vi "Do_channel_maths.vi"(4 "Output Index":i32, 5 "Channel Values In":string[][](array[string]), 6 "Channel Names":string[](array[string]), 7 "Maths Equation":string) -> (0 "Error String":string, 1 "Channel Values Out":string[][](array[string]), 3 "Results":dbl[](array[numeric]) format="%0.2f")   [LabVIEW 2021]
uses:
  Data_plotting_vis/Results_plotter_Global.vi
  <vilib>/gmath/NI_Gmath.lvlib
panel:
  out "Numeric":i32
  out "AuditTrail":string[](array[string])
  out "Generic Equation":string
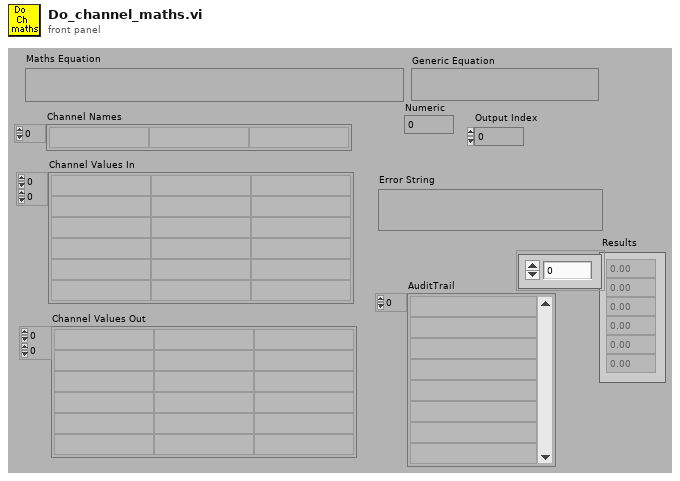
[diagram p1: front panel]
types:
  T1 = cluster{"Tables":i32[][], "Y Values":dbl[], "Variables input decode":i32[], i32[]}[]
  T2 = cluster{"Y Values":dbl[][], "Tables":i32[][][], "Variables input decode":i32[], "Variables output decode":i32[]}
  T3 = cluster{"Tables":i32[][], "Y Values":dbl[], "Variables input decode":i32[], i32[]}
  T4 = typedef "LVDateTimeRec.ctl" = cluster{"fractional second":dbl, "second":i32, "minute":i32, "hour":i32, "day of month":i32, "month":i32, "year":i32, "day of week":i32, "day of year":i32, "DST":i32}
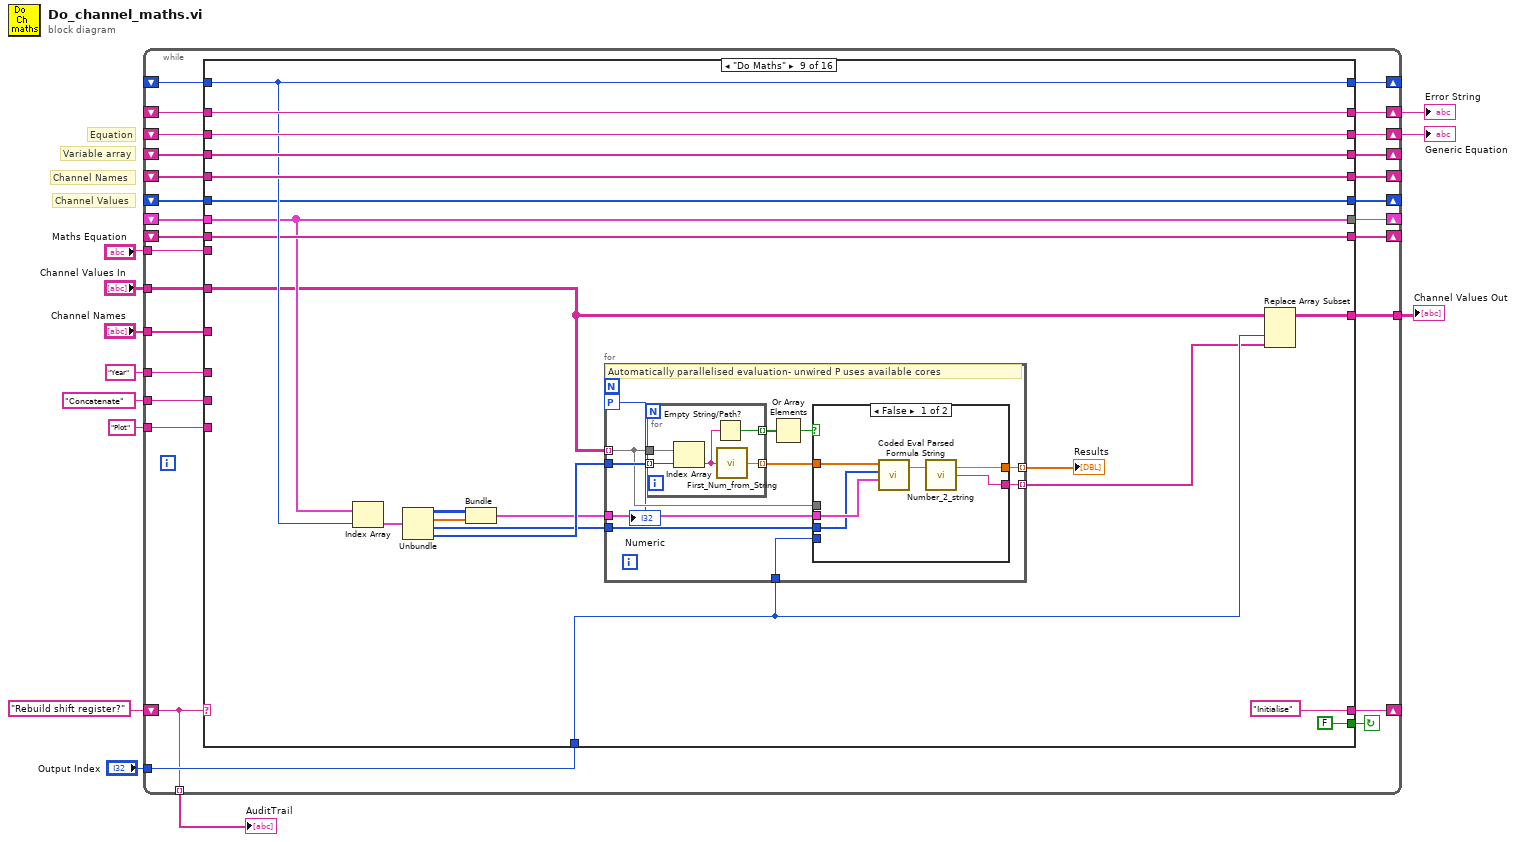
[diagram p0: block diagram]
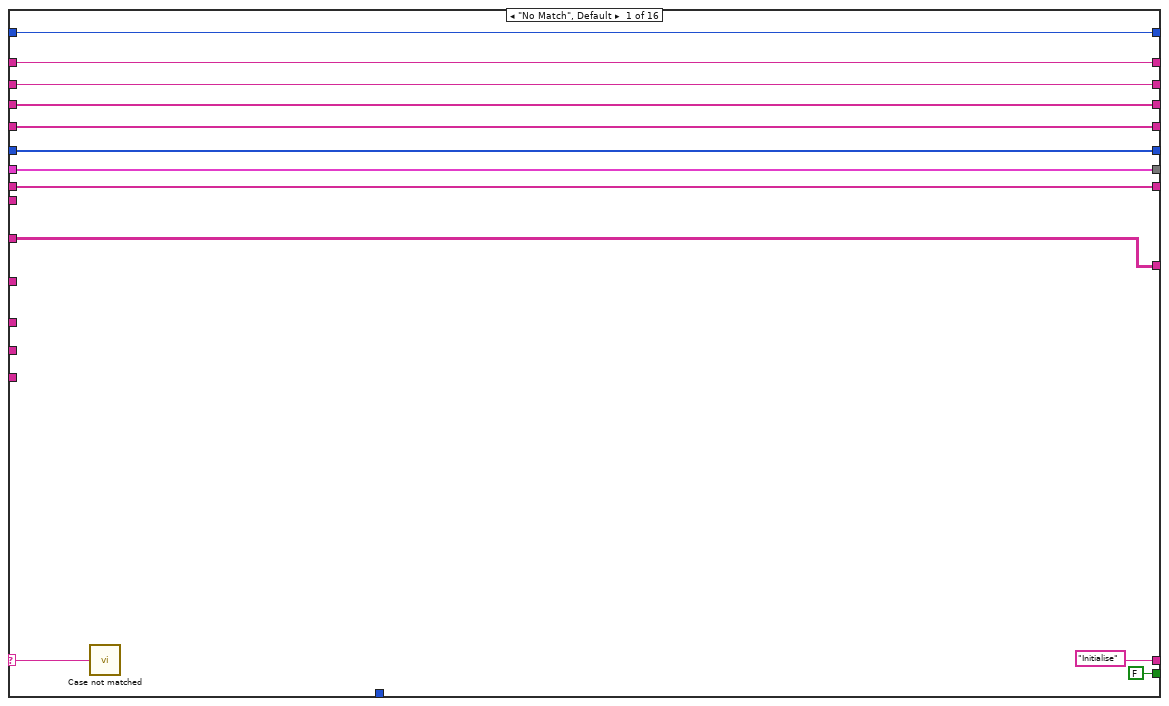
[diagram p2: hidden frame]
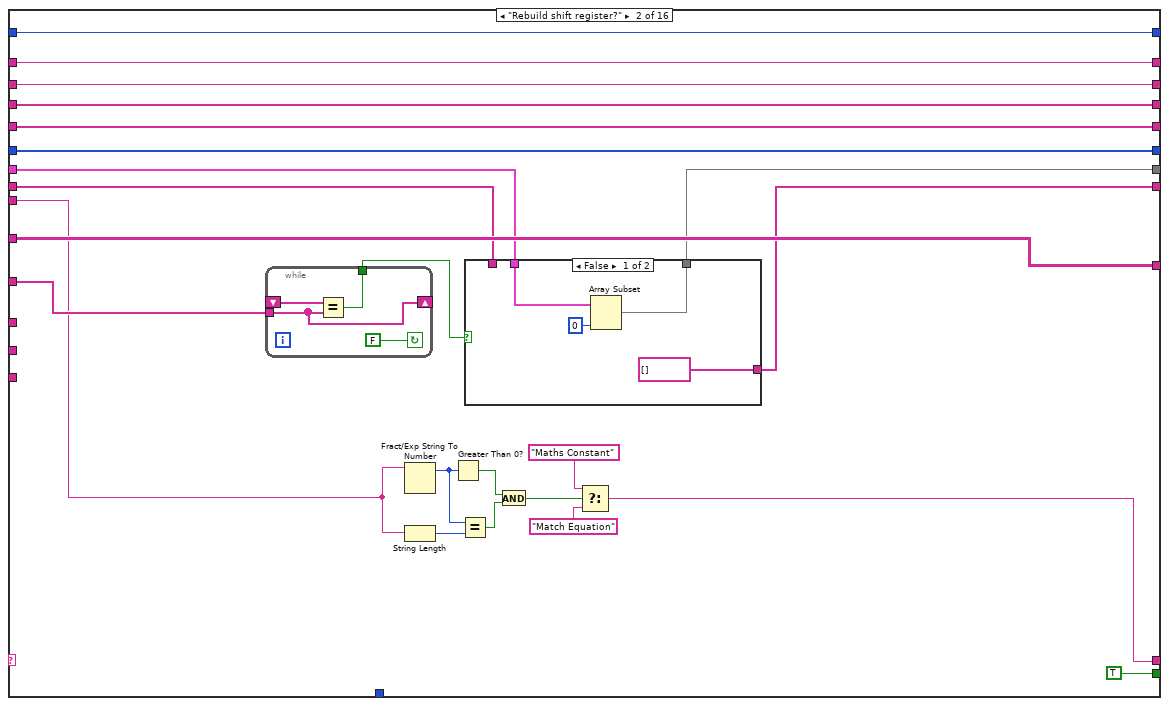
[diagram p3: hidden frame]
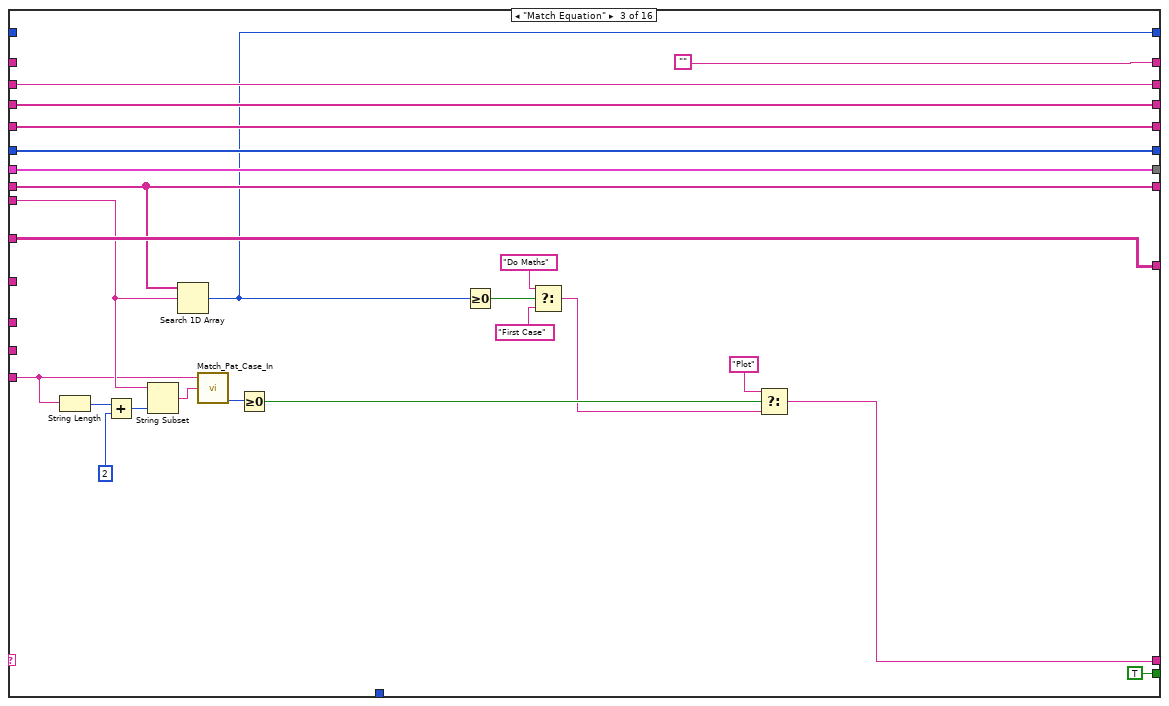
[diagram p5: hidden frame]
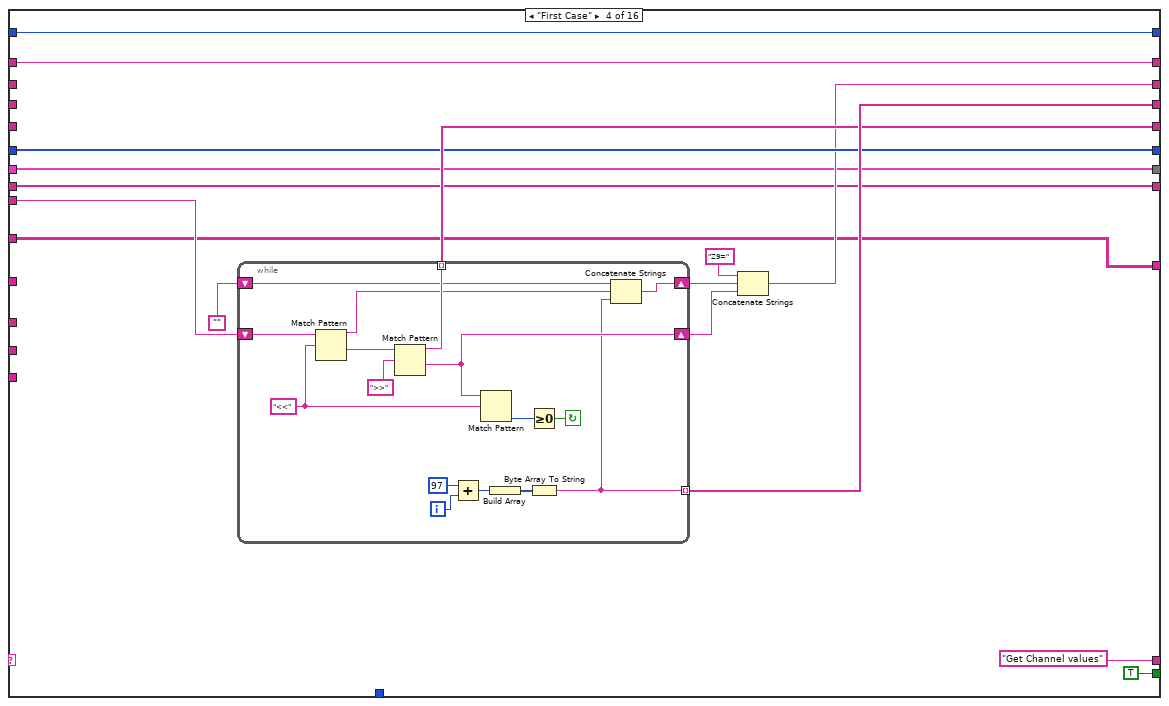
[diagram p6: hidden frame]
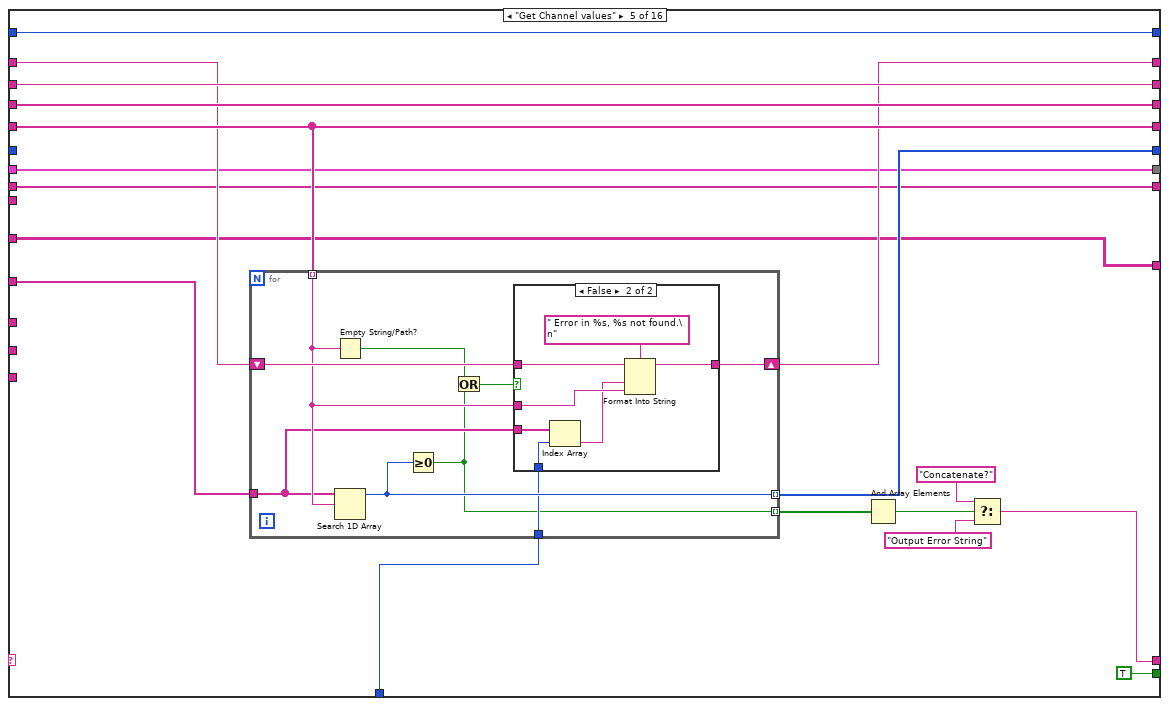
[diagram p7: hidden frame]
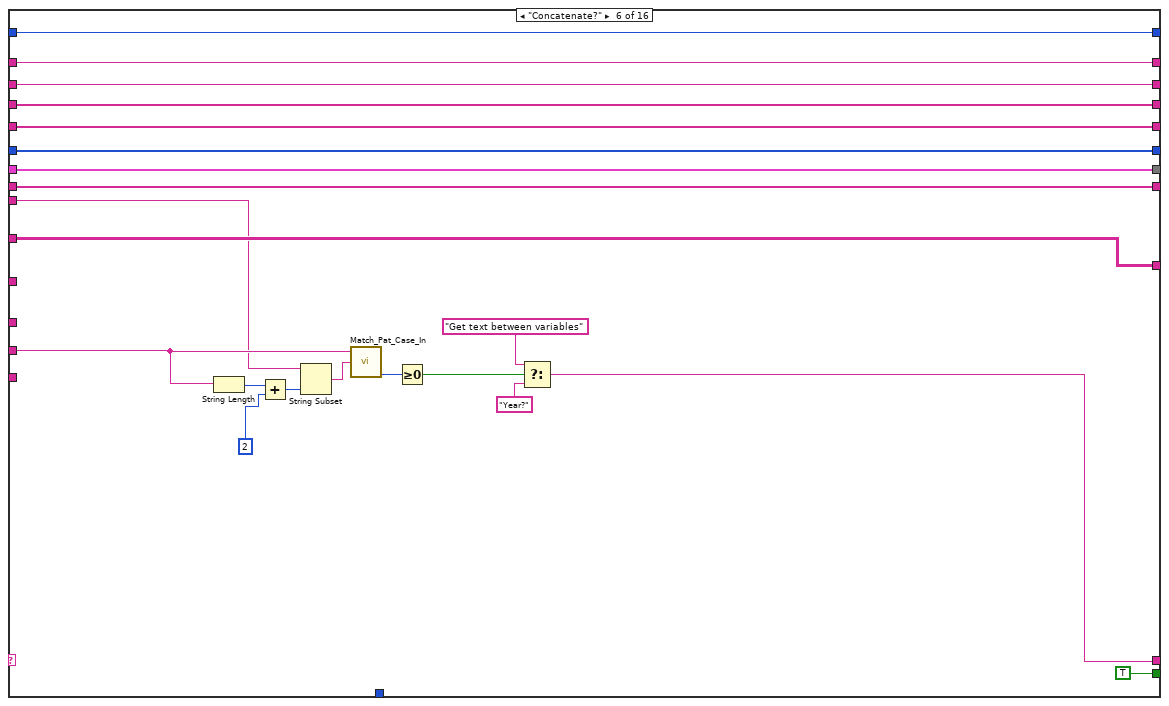
[diagram p9: hidden frame]
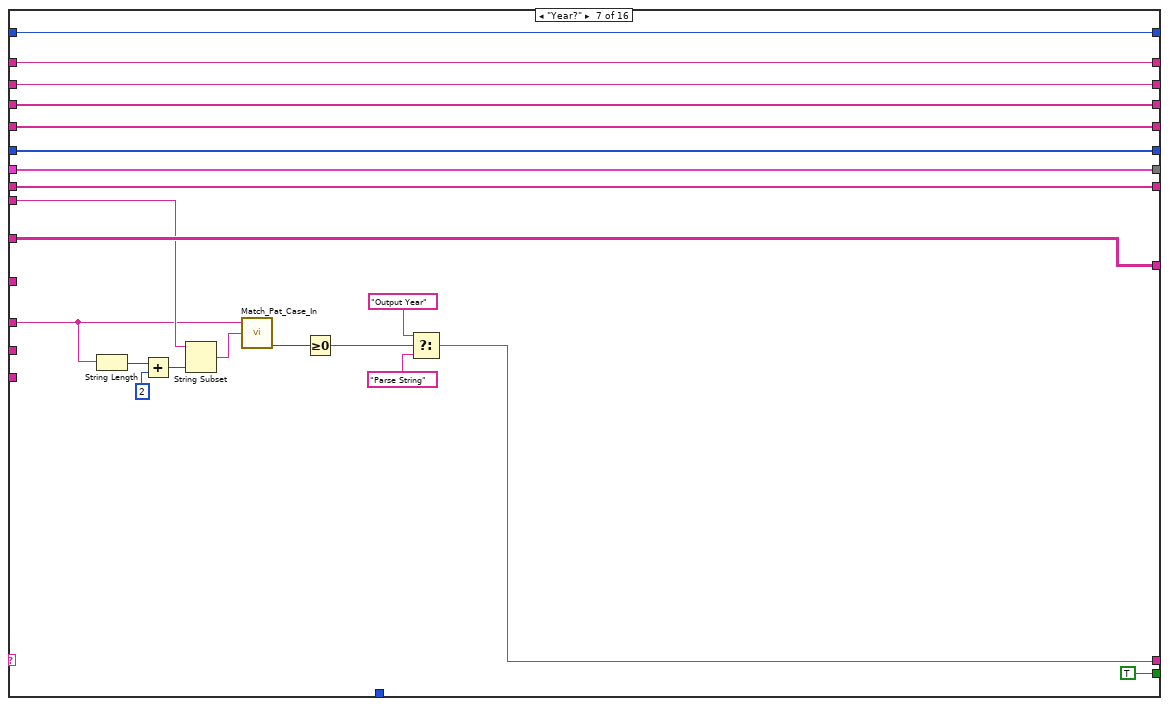
[diagram p10: hidden frame]
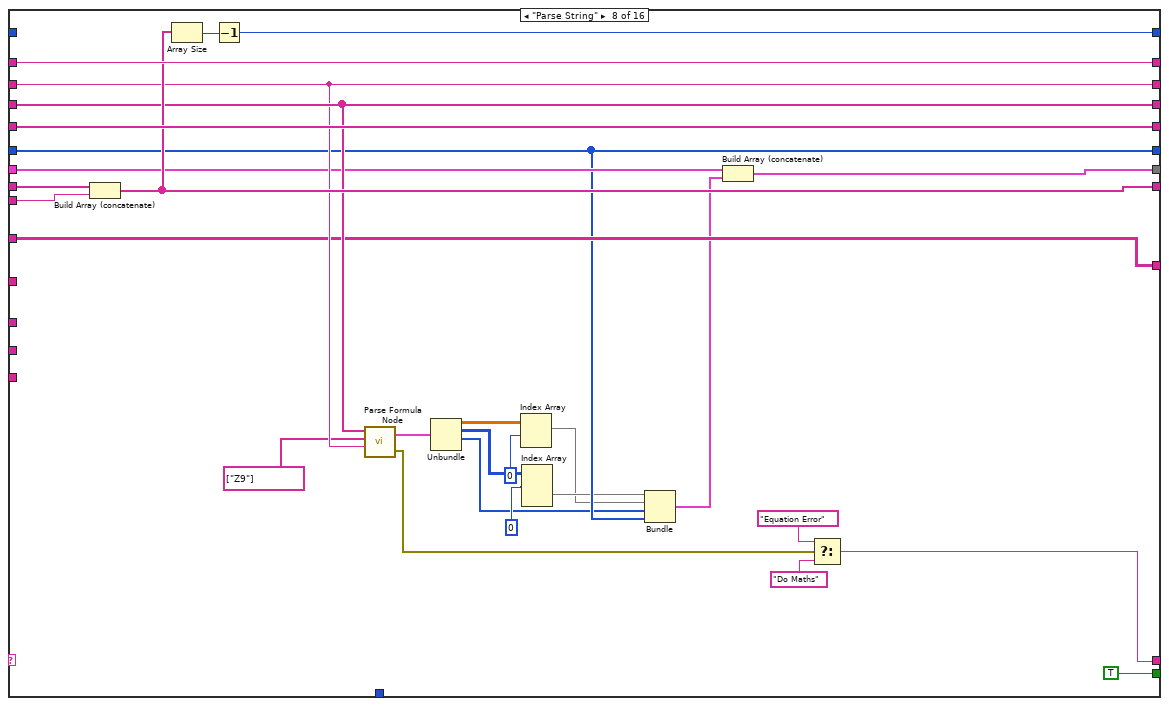
[diagram p11: hidden frame]
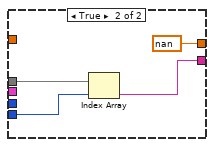
[diagram p12: hidden frame]
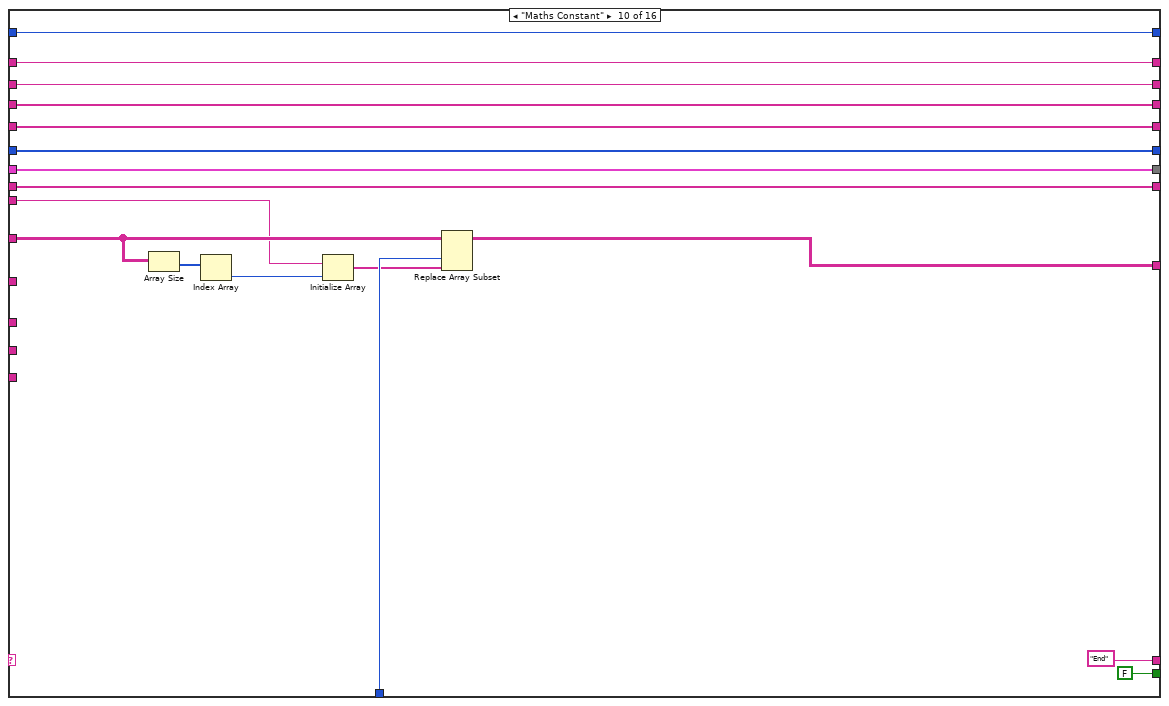
[diagram p13: hidden frame]
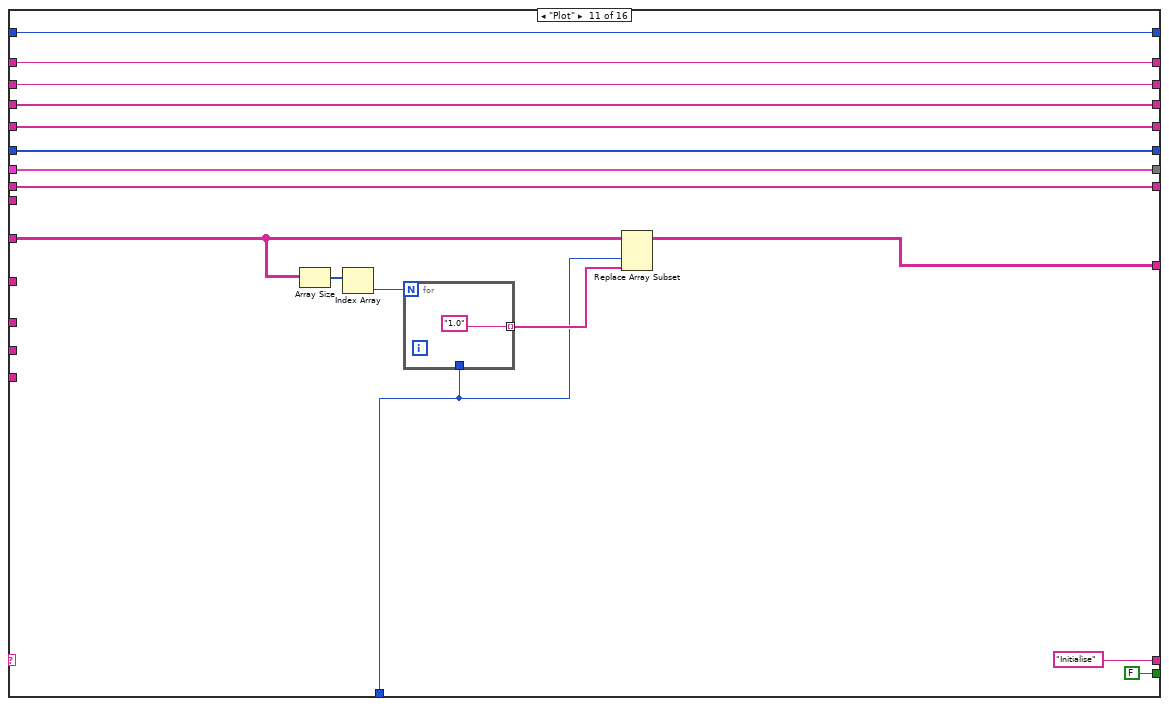
[diagram p14: hidden frame]
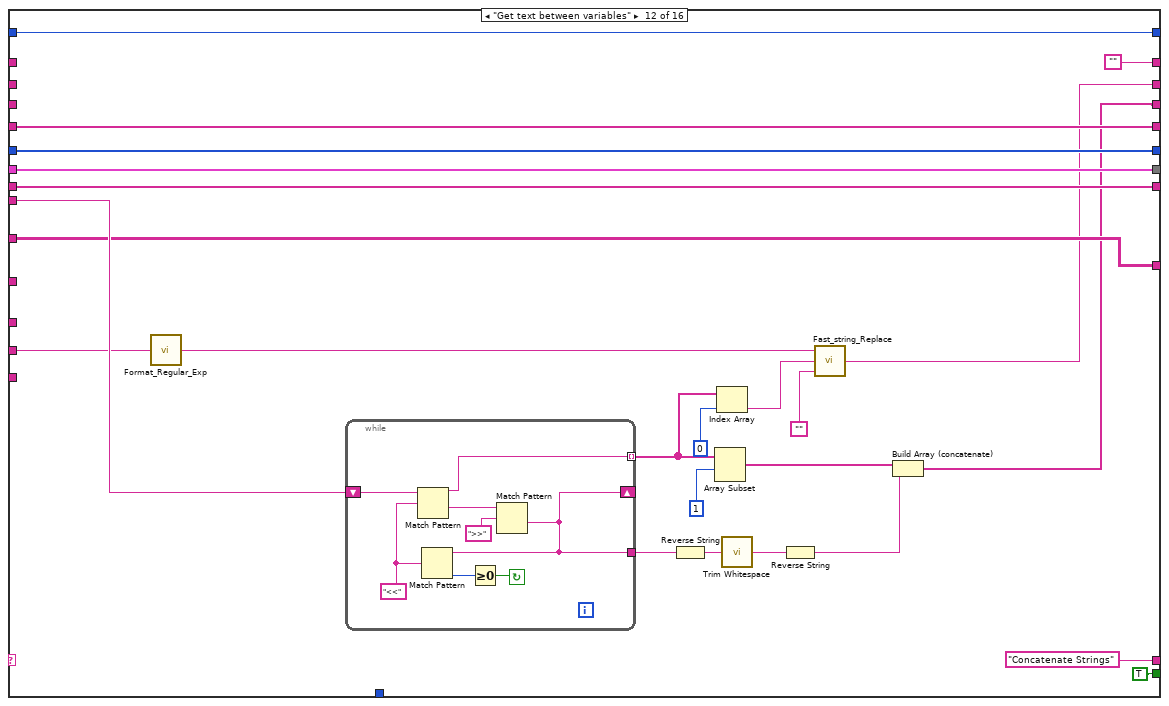
[diagram p15: hidden frame]
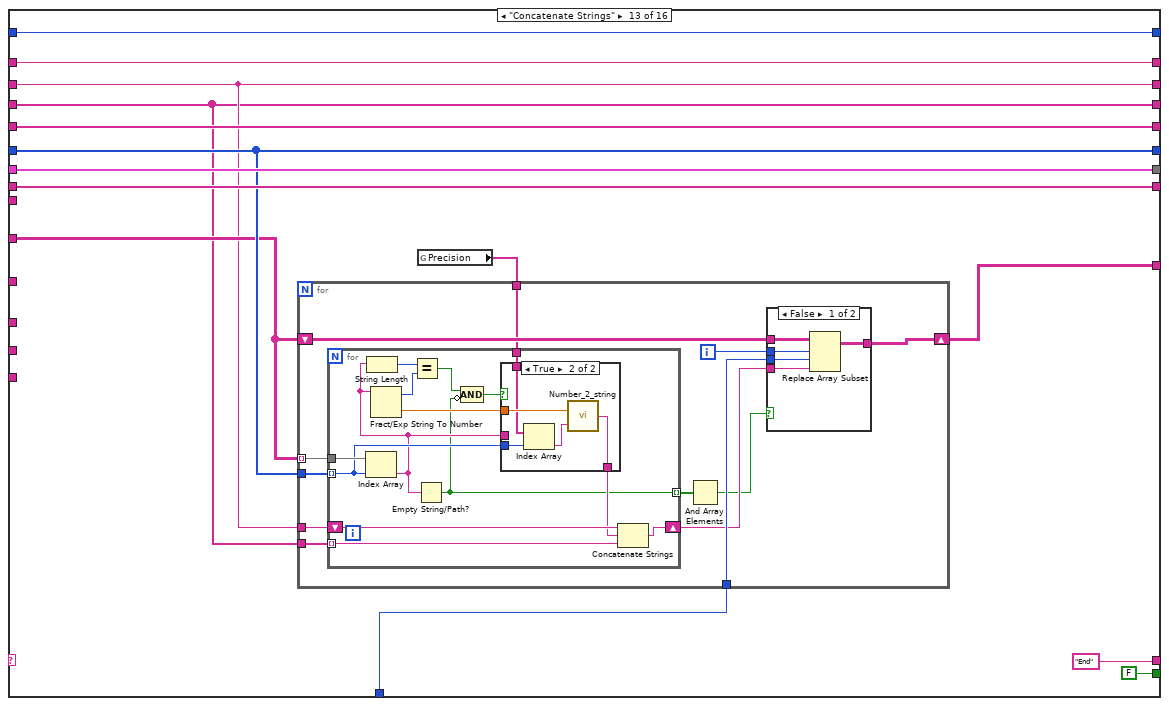
[diagram p16: hidden frame]
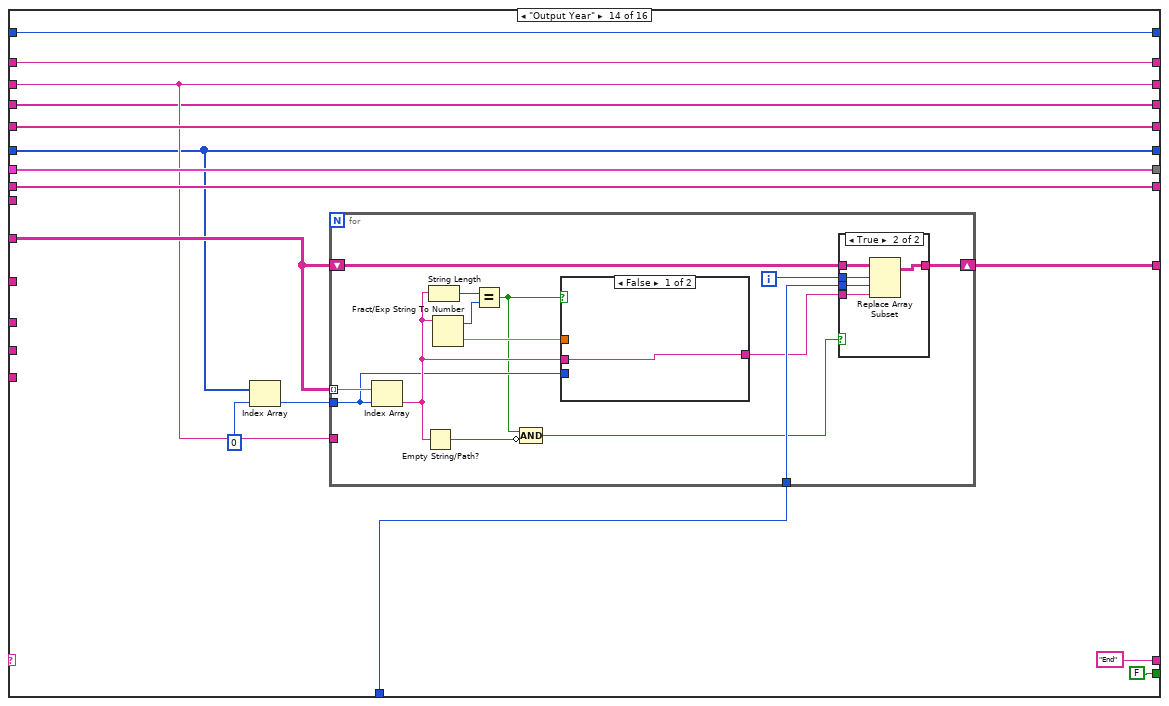
[diagram p19: hidden frame]
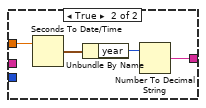
[diagram p20: hidden frame]
diagram:
  # "Channel Names"
  # "Variable array"
  # "Channel Values"
  # "Equation"
  n1 = while {
    tunnel: [w17] -> w6
    tunnel: "Output Index" -> [w18]
    shift-left: _ -> [w19]
    shift-right: [w20] -> _
    shift-left: _ -> [w23]
    shift-right: [w22] -> _
    shift-left: _ -> [w21]
    shift-right: [w24] -> _
    tunnel: "Channel Values In" -> [w25]
    tunnel: "Channel Names" -> [w26]
    tunnel: "Maths Equation" -> [w27]
    shift-left: _ -> [w29]
    shift-right: [w28] -> _
    shift-left: _ -> [w31]
    shift-right: [w30] -> _
    shift-left: _ -> [w33]
    shift-right: [w32] -> _
    shift-left: _ -> [w35]
    shift-right: [w34] -> w8
    shift-left: _ -> [w37]
    shift-right: [w36] -> w9
    shift-left: "Rebuild shift register?" -> [w13]
    shift-right: [w38] -> _
    tunnel: "Concatenate" ("regular expression") -> [w16]
    tunnel: "Plot" ("regular expression") -> [w15]
    tunnel: "Year" ("regular expression") -> [w14]
    tunnel: [w13] -> w1 mode=indexing
    stop <- w39 continue-if-true
    n2 = case shown="\"Do Maths\"" w13 {
      selector: w13 -> [w40 _ _ _ _ _ _ _ _ _ _ _ _ _ _ _]
      tunnel: [FALSE TRUE TRUE TRUE TRUE TRUE TRUE TRUE FALSE FALSE FALSE TRUE FALSE FALSE TRUE FALSE] -> w39
      tunnel: ["Initialise" w53 w86 "Get Channel values" w143 w176 w206 w232 "Initialise" "End" "Initialise" "Concatenate Strings" "End" "End" "Output Error String" "Initialise"] -> w38
      tunnel: w37 -> [w49 w73 _ w109 w151 w196 w217 w243 w263 w305 w321 _ w368 w421 w451 w464]
      tunnel: [w49 w73 "" w109 w152 w196 w217 w243 w263 w305 w321 "" w368 w421 w450 w464] -> w36
      tunnel: w35 -> [w48 w72 w108 _ w157 w195 w216 w239 w261 w303 w319 _ w360 w414 w453 w474]
      tunnel: [w48 w72 w108 w114 w157 w195 w216 w239 w261 w303 w319 w335 w360 w414 w453 w474] -> w34
      tunnel: w33 -> [w47 w71 w107 _ w156 w194 w215 w240 w262 w304 w320 _ w359 w413 w460 w475]
      tunnel: [w47 w71 w107 w121 w156 w194 w215 w240 w262 w304 w320 w330 w359 w413 w460 w475] -> w32
      tunnel: w31 -> [w46 w70 w106 _ w154 w193 w214 w244 w264 w306 w322 w340 w369 w422 w461 w476]
      tunnel: [w46 w70 w106 w117 w154 w193 w214 w244 w264 w306 w322 w340 w369 w422 w461 w476] -> w30
      tunnel: w29 -> [w45 w69 w105 w116 _ w192 w213 w231 w254 w299 w315 w345 w364 w412 w456 w468]
      tunnel: [w45 w69 w105 w116 w153 w192 w213 w231 w254 w299 w315 w345 w364 w412 w456 w468] -> w28
      tunnel: w27 -> [_ w52 w92 w122 _ w180 w200 w218 _ w293 _ w347 _ _ w452 _]
      tunnel: w26 -> [_ w66 _ _ w155 _ _ _ _ _ _ _ _ _ _ w466]
      tunnel: w25 -> [w41 w67 w103 w110 w147 w187 w205 w235 w252 w296 w311 w341 w363 w417 w455 w467]
      tunnel: [w44 w64 w104 w113 w150 w191 w212 w236 w258 w300 w316 w344 w365 w418 w457 w471] -> w24
      tunnel: w23 -> [w43 w62 w102 w112 w149 w190 w211 w242 w259 w301 w317 w343 w366 w419 w458 w472]
      tunnel: [w43 w61 w102 w112 w149 w190 w211 w241 w259 w301 w317 w343 w366 w419 w458 w472] -> w22
      tunnel: w21 -> [w44 w63 w104 w113 w150 w191 w212 w238 w258 w300 w316 w344 w365 w418 w457 w471]
      tunnel: [w42 w68 w101 w111 w148 w189 w210 w237 w260 w302 w318 w342 w367 w420 w459 w473] -> w20
      tunnel: w19 -> [w42 w68 _ w111 w148 w189 w210 _ w260 w302 w318 w342 w367 w420 w459 w473]
      tunnel: w18 -> [_ _ _ _ w141 _ _ _ w251 w297 w312 _ w362 w416 _ w470]
      tunnel: [w41 w67 w103 w110 w147 w187 w205 w235 w253 w298 w314 w341 w361 w415 w455 w469] -> w17
      tunnel: w16 -> [_ _ _ _ _ w186 _ _ _ _ _ w337 _ _ _ _]
      tunnel: w15 -> [_ _ w91 _ _ _ _ _ _ _ _ _ _ _ _ _]
      tunnel: w14 -> [_ _ _ _ _ _ w197 _ _ _ _ _ _ _ _ _]
      frame "No Match", Default {
        n3 = call "Case not matched.vi"("Case Name not Matched"=w40) -> ()
      }
      frame "Rebuild shift register?" {
        n4 = while {
          shift-right: [w83] -> _
          shift-left: _ -> [w84]
          tunnel: w66 -> [w83]
          tunnel: [w82] -> w65
          stop <- FALSE continue-if-true
          n5 = Equal?(x=w84, y=w83) -> (x = y?=w82:bool)
        }
        n6 = Fract/Exp String To Number(string=w52) -> (offset past number=w60:i32)  [unwired: 3 in, 1 out]
        n7 = String Length(string=w52) -> (length=w59:i32)
        n8 = Greater Than 0?(x=w60) -> (x > 0?=w57:bool)
        n9 = Equal?(x=w60, y=w59) -> (x = y?=w58:bool)
        n10 = case shown="False" w65 {
          tunnel: [w76 w80] -> w64
          tunnel: w63 -> [w78 w80]
          tunnel: w62 -> [_ w79]
          tunnel: [string[] [] w79] -> w61
          frame False {
            n11 = Array Subset(array=w78, length=0) -> (w76:T1)  [unwired: 1 in]
          }
          frame True {
          }
        }
        n12 = And(x=w57, y=w58) -> (x .and. y?=w56:bool)
        n13 = Select(t="Maths Constant", s=w56, f="Match Equation") -> (s? t:f=w53:string)
      }
      frame "Match Equation" {
        n14 = String Length(string=w91) -> (length=w93:i32)
        n15 = Add(x=w93, y=2) -> (x+y=w95:i32)
        n16 = String Subset(string=w92, length (rest)=w95) -> (substring=w96:string)  [unwired: 1 in]
        n17 = Search 1D Array(1D array=w102, element=w92) -> (index of element=w101:i32)  [unwired: 1 out]
        n18 = call "Match_Pat_Case_In.vi"("String to match"=w91, "String"=w96) -> ("offset past match"=w89:i32)  [unwired: 1 in, 3 out]
        n19 = Greater Or Equal To 0?(x=w89) -> (x >= 0?=w88:bool)
        n20 = Greater Or Equal To 0?(x=w101) -> (x >= 0?=w100:bool)
        n21 = Select(t="Do Maths", s=w100, f="First Case") -> (s? t:f=w87:string)
        n22 = Select(t="Plot", s=w88, f=w87) -> (s? t:f=w86:string)
      }
      frame "First Case" {
        n23 = while {
          shift-left: "" -> [w127]
          shift-right: [w128] -> w119
          tunnel: [w129] -> w121 mode=indexing
          tunnel: [w135] -> w117 mode=indexing
          shift-left: w122 -> [w140]
          shift-right: [w138] -> w118
          i -> [w131]
          stop <- w136 continue-if-true
          w126 = "<<" ("regular expression")
          n24 = Match Pattern(string=w140, regular expression=w126) -> (before substring=w130:string, after substring=w139:string)  [unwired: 3 out]
          n25 = Match Pattern(string=w139, regular expression=">>") -> (before substring=w135:string, after substring=w138:string)  [unwired: 3 out]
          n26 = Add(x=97, y=w131) -> (x+y=w133:i32)
          n27 = Match Pattern(string=w138, regular expression=w126) -> (offset past match=w137:i32)  [unwired: 4 out]
          n28 = Build Array(w133) -> (w134:i32[])
          n29 = Greater Or Equal To 0?(x=w137) -> (x >= 0?=w136:bool)
          n30 = Byte Array To String(unsigned byte array=w134) -> (string=w129:string)
          n31 = Concatenate Strings(w127, w130, w129) -> (w128:string)
        }
        n32 = Concatenate Strings("Z9=" ("Substring"), w119, w118) -> (w114:string)
      }
      frame "Get Channel values" {
        n33 = for {
          tunnel: w155 -> [w162]
          tunnel: w154 -> [w164] mode=indexing
          tunnel: [w165] -> w153 mode=indexing
          shift-right: [w166] -> w152
          shift-left: w151 -> [w167]
          tunnel: [w159] -> w146 mode=indexing
          tunnel: w141 -> [w161]
          n34 = Empty String/Path?(string/path=w164) -> (empty?=w160:bool)
          n35 = Search 1D Array(1D array=w162, element=w164) -> (index of element=w165:i32)  [unwired: 1 out]
          n36 = Greater Or Equal To 0?(x=w165) -> (x >= 0?=w159:bool)
          n37 = Or(x=w160, y=w159) -> (x .or. y?=w163:bool)
          n38 = case shown="False" w163 {
            tunnel: w164 -> [_ w175]
            tunnel: w167 -> [w168 w173]
            tunnel: [w168 w172] -> w166
            tunnel: w162 -> [_ w171]
            tunnel: w161 -> [_ w170]
            frame True {
            }
            frame False {
              n39 = Index Array(array=w171, index=w170) -> (element=w169:string)
              n40 = Format Into String(format string=" Error in %s, %s not found.\n" ("Format String"), initial string=w173, w169, w175) -> (resulting string=w172:string)  [unwired: 1 in, 1 out]
            }
          }
        }
        n41 = And Array Elements(Boolean array=w146) -> (logical AND=w145:bool)
        n42 = Select(t="Concatenate?", s=w145, f="Output Error String") -> (s? t:f=w143:string)
      }
      frame "Concatenate?" {
        n43 = String Length(string=w186) -> (length=w185:i32)
        n44 = Add(x=w185, y=2) -> (x+y=w183:i32)
        n45 = String Subset(string=w180, length (rest)=w183) -> (substring=w182:string)  [unwired: 1 in]
        n46 = call "Match_Pat_Case_In.vi"("String to match"=w186, "String"=w182) -> ("offset past match"=w188:i32)  [unwired: 1 in, 3 out]
        n47 = Greater Or Equal To 0?(x=w188) -> (x >= 0?=w178:bool)
        n48 = Select(t="Get text between variables" ("regular expression"), s=w178, f="Year?" ("regular expression")) -> (s? t:f=w176:string)
      }
      frame "Year?" {
        n49 = String Length(string=w197) -> (length=w204:i32)
        n50 = Add(x=w204, y=2) -> (x+y=w202:i32)
        n51 = String Subset(string=w200, length (rest)=w202) -> (substring=w201:string)  [unwired: 1 in]
        n52 = call "Match_Pat_Case_In.vi"("String to match"=w197, "String"=w201) -> ("offset past match"=w209:i32)  [unwired: 1 in, 3 out]
        n53 = Greater Or Equal To 0?(x=w209) -> (x >= 0?=w199:bool)
        n54 = Select(t="Output Year" ("regular expression"), s=w199, f="Parse String" ("regular expression")) -> (s? t:f=w206:string)
      }
      frame "Parse String" {
        n55 = Build Array (concatenate)(w242, w218) -> (w241:string[])
        n56 = Array Size(array=w241) -> (size(s)=w229:i32)
        n57 = Decrement(x=w229) -> (x-1=w237:i32)
        n58 = call <vilib>:"Parse Formula Node.vi"("formula"=w239, "Variables Output"=string[] ["Z9"], "Variables Input"=w240) -> ("error out"=w219:errorcluster, "Parsed Formula Node"=w228:T2)  [unwired: 1 in]
        n59 = Unbundle(w228) -> ("Y Values"=w227:dbl[][], "Tables"=w224:i32[][][], "Variables input decode"=w221:i32[])  [unwired: 1 out]
        n60 = Index Array(array=w227, index (row)=0 ("Index")) -> (element=w222:dbl[])  [unwired: 1 in]
        n61 = Index Array(array=w224, index (dim 0)=0 ("Index")) -> (element=w223:i32[][])  [unwired: 2 in]
        n62 = Bundle("Tables"=w223, "Y Values"=w222, "Variables input decode"=w221, w231) -> (w220:T3)  [unwired: 1 out]
        n63 = Build Array (concatenate)(w238, w220) -> (w236:T1)
        n64 = Select(t="Equation Error", s=w219, f="Do Maths") -> (s? t:f=w232:string)
      }
      frame "Do Maths" {
        n65 = Index Array(array=w258, index=w260) -> (element=w257:T3)
        n66 = Unbundle(w257) -> ("Tables"=w256:i32[][], "Y Values"=w255:dbl[], "Variables input decode"=w249:i32[], w250:i32[])
        n67 = Bundle("Tables"=w256, "Y Values"=w255) -> (w248:cluster{"Tables":i32[][], "Y Values":dbl[]})  [unwired: 1 out]
        n68 = for {
          tunnel: w252 -> [w270] mode=indexing
          tunnel: w250 -> [w277]
          tunnel: w248 -> [w275]
          tunnel: w249 -> [w274]
          tunnel: [w271] -> w247 mode=indexing
          tunnel: w251 -> [w269]
          tunnel: [w268] -> w246 mode=indexing
          workers-P: _ -> [w267]
          # "Automatically parallelised evaluation- unwired P uses available cores"
          n69 = for {
            tunnel: w270 -> [w291]
            tunnel: w277 -> [w290] mode=indexing
            tunnel: [w287] -> w276 mode=indexing
            tunnel: [w289] -> w273 mode=indexing
            n70 = Index Array(array=w291, index=w290) -> (element=w288:string)
            n71 = Empty String/Path?(string/path=w288) -> (empty?=w289:bool)
            n72 = call "First_Num_from_String.vi"("string"=w288) -> ("number"=w287:dbl)
          }
          n73 = Or Array Elements(Boolean array=w273) -> (logical OR=w272:bool)
          n74 = case shown="False" w272 {
            tunnel: w276 -> [w282 _]
            tunnel: w275 -> [w281 _]
            tunnel: w274 -> [w280 _]
            tunnel: [w279 w284] -> w271
            tunnel: w270 -> [_ w286]
            tunnel: w269 -> [_ w285]
            tunnel: [w278 nan ("y value")] -> w268
            frame False {
              n75 = call <vilib>:"Coded Eval Parsed Formula String.vi"("Parsed Formula"=w281, "Variables"=w280, "X Values"=w282) -> ("y value"=w278:dbl)  [unwired: 1 in, 1 out]
              n76 = call "Number_2_string.vi"("number"=w278) -> ("String"=w279:string)  [unwired: 1 in]
            }
            frame True {
              n77 = Index Array(array=w286, index=w285) -> (element=w284:string)
            }
          }
          "Numeric" <- w267
        }
        "Results" <- w246
        n78 = Replace Array Subset(array=w252, new element=w247, index (col)=w251) -> (w253:string[][])  [unwired: 1 in]
      }
      frame "Maths Constant" {
        n79 = Array Size(array=w296) -> (size(s)=w295:i32[])
        n80 = Index Array(array=w295) -> (element=w294:i32)  [unwired: 1 in]
        n81 = Initialize Array(w293, w294) -> (w292:string[])
        n82 = Replace Array Subset(array=w296, new element=w292, index (col)=w297) -> (w298:string[][])  [unwired: 1 in]
      }
      frame "Plot" {
        n83 = Array Size(array=w311) -> (size(s)=w310:i32[])
        n84 = Index Array(array=w310) -> (element=w309:i32)  [unwired: 1 in]
        n85 = for {
          N: w309 -> [_]
          tunnel: ["1.0"] -> w313 mode=indexing
          tunnel: w312 -> [_]
        }
        n86 = Replace Array Subset(array=w311, new element=w313, index (col)=w312) -> (w314:string[][])  [unwired: 1 in]
      }
      frame "Get text between variables" {
        n87 = call "Format_Regular_Exp.vi"("Regular expression"=w337) -> ("Case Insensitive for html"=w336:string)
        n88 = while {
          shift-left: w347 -> [w357]
          shift-right: [w352] -> _
          tunnel: [w353] -> w333 mode=indexing
          tunnel: [w352] -> w329
          stop <- w354 continue-if-true
          w351 = "<<" ("regular expression")
          n89 = Match Pattern(string=w357, regular expression=w351) -> (before substring=w353:string, after substring=w356:string)  [unwired: 3 out]
          n90 = Match Pattern(string=w356, regular expression=">>") -> (after substring=w352:string)  [unwired: 4 out]
          n91 = Match Pattern(string=w352, regular expression=w351) -> (offset past match=w355:i32)  [unwired: 4 out]
          n92 = Greater Or Equal To 0?(x=w355) -> (x >= 0?=w354:bool)
        }
        n93 = Reverse String(1:w329) -> (0:w328:string)
        n94 = Array Subset(array=w333, index=1) -> (w332:string[])  [unwired: 1 in]
        n95 = Index Array(array=w333, index=0) -> (element=w338:string)
        n96 = call <vilib>:"Trim Whitespace.vi"("string"=w328) -> ("trimmed string"=w327:string)  [unwired: 1 in]
        n97 = Reverse String(1:w327) -> (0:w326:string)
        n98 = call "Fast_string_Replace.vi"("Replace match with:"="", "Input String"=w338, "regular expression"=w336) -> ("Output String"=w335:string)  [unwired: 2 out]
        n99 = Build Array (concatenate)(w332, w326) -> (w330:string[])
      }
      frame "Concatenate Strings" {
        n100 = global read "Results_plotter_Global.vi" "Precision"() -> (w358:string[])
        n101 = for {
          tunnel: w363 -> [w383] mode=indexing
          shift-right: [w380] -> w361
          shift-left: w363 -> [w381]
          tunnel: w364 -> [w382]
          tunnel: w362 -> [w378]
          tunnel: w360 -> [w377]
          tunnel: w359 -> [w376]
          tunnel: w358 -> [w375]
          i -> [w379]
          n102 = for {
            tunnel: w383 -> [w403]
            tunnel: w382 -> [w396] mode=indexing
            shift-right: [w394] -> w374
            shift-left: w377 -> [w402]
            tunnel: w376 -> [w401] mode=indexing
            tunnel: w375 -> [w395]
            tunnel: [w391] -> w373 mode=indexing
            n103 = Index Array(array=w403, index=w396) -> (element=w393:string)
            n104 = String Length(string=w393) -> (length=w400:i32)
            n105 = Fract/Exp String To Number(string=w393) -> (offset past number=w399:i32, number=w398:dbl)  [unwired: 3 out]
            n106 = Equal?(x=w400, y=w399) -> (x = y?=w392:bool)
            n107 = Empty String/Path?(string/path=w393) -> (empty?=w391:bool)
            n108 = Compound Arithmetic op=AND(w392, invert w391) -> (w390:bool)
            n109 = case shown="True" w390 {
              tunnel: w398 -> [_ w409]
              tunnel: [w404 w408] -> w397
              tunnel: w393 -> [w404 _]
              tunnel: w396 -> [_ w407]
              tunnel: w395 -> [_ w406]
              frame False {
              }
              frame True {
                n110 = Index Array(array=w406, index=w407) -> (element=w405:string)
                n111 = call "Number_2_string.vi"("precision"=w405, "number"=w409) -> ("String"=w408:string)
              }
            }
            n112 = Concatenate Strings(w402, w397, w401) -> (w394:string)
          }
          n113 = And Array Elements(Boolean array=w373) -> (logical AND=w372:bool)
          n114 = case shown="False" w372 {
            tunnel: w381 -> [w388 w389]
            tunnel: [w387 w389] -> w380
            tunnel: w379 -> [w386 _]
            tunnel: w378 -> [w385 _]
            tunnel: w374 -> [w384 _]
            frame False {
              n115 = Replace Array Subset(array=w388, new element=w384, index (row)=w386, index (col)=w385) -> (w387:string[][])
            }
            frame True {
            }
          }
        }
      }
      frame "Output Year" {
        n116 = Index Array(array=w412, index=0) -> (element=w410:i32)
        n117 = for {
          tunnel: w417 -> [w438] mode=indexing
          shift-right: [w436] -> w415
          shift-left: w417 -> [w437]
          tunnel: w416 -> [w434]
          tunnel: w414 -> [_]
          tunnel: w410 -> [w429]
          i -> [w435]
          n118 = Index Array(array=w438, index=w429) -> (element=w430:string)
          n119 = Empty String/Path?(string/path=w430) -> (empty?=w427:bool)
          n120 = String Length(string=w430) -> (length=w433:i32)
          n121 = Fract/Exp String To Number(string=w430) -> (offset past number=w432:i32, number=w431:dbl)  [unwired: 3 out]
          n122 = Equal?(x=w433, y=w432) -> (x = y?=w426:bool)
          n123 = Compound Arithmetic op=AND(w426, invert w427) -> (w425:bool)
          n124 = case shown="False" w426 {
            tunnel: w431 -> [_ w443]
            tunnel: [w439 w440] -> w428
            tunnel: w430 -> [w439 _]
            tunnel: w429 -> [_ _]
            frame False {
            }
            frame True {
              n125 = Seconds To Date/Time(time stamp (now)=w443) -> (date time rec=w442:T4)  [unwired: 1 in]
              n126 = Unbundle By Name(w442) -> ("year"=w441:i32)
              n127 = Number To Decimal String(number=w441) -> (decimal integer string=w440:string)  [unwired: 1 in]
            }
          }
          n128 = case shown="True" w425 {
            tunnel: w437 -> [w444 w449]
            tunnel: [w444 w448] -> w436
            tunnel: w435 -> [_ w447]
            tunnel: w434 -> [_ w446]
            tunnel: w428 -> [_ w445]
            frame False {
            }
            frame True {
              n129 = Replace Array Subset(array=w449, new element=w445, index (row)=w447, index (col)=w446) -> (w448:string[][])
            }
          }
        }
      }
      frame "Equation Error" {
        n130 = Format Into String(format string="There is an error in the Maths Equation %s. The full equation is %s", initial string=w451, w453, w452) -> (resulting string=w450:string)  [unwired: 1 in, 1 out]
      }
      frame "Output Error String" {
        n131 = Array Size(array=w466) -> (size(s)=w465:i32)
        n132 = for {
          N: w465 -> [_]
          shift-right: [w482] -> w469
          shift-left: w467 -> [w483]
          tunnel: w470 -> [w480]
          tunnel: w464 -> [w479]
          i -> [w481]
          n133 = Replace Array Subset(array=w483, new element=w479, index (row)=w481, index (col)=w480) -> (w482:string[][])
        }
      }
    }
  }
  "Error String" <- w9
  "Generic Equation" <- w8
  "Channel Values Out" <- w6
  "AuditTrail" <- w1
